vi "Write APD Serial.vi"(8 "error in (no error)":errorcluster, 10 "APD Serial #":string, 11 "APDClass in":refnum<class "APDClass.lvclass">) -> (0 "error out":errorcluster, 3 "APDClass out":refnum<class "APDClass.lvclass">)   [LabVIEW 2020, in "APDClass.lvclass"]
uses:
  APDClass.lvclass
  APDClass.lvclass/APDClass.ctl
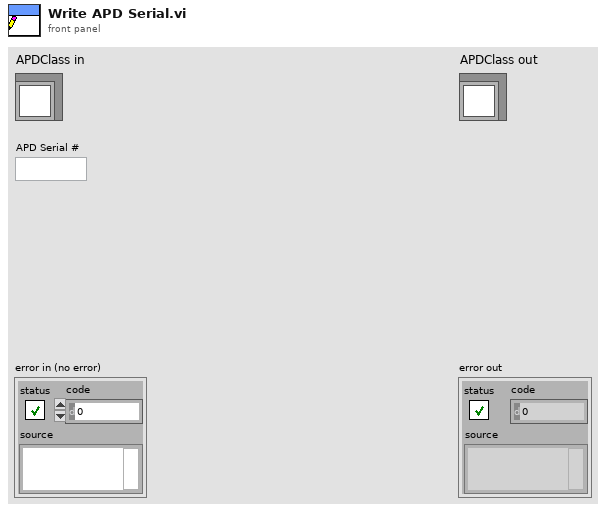
[diagram p1: front panel]
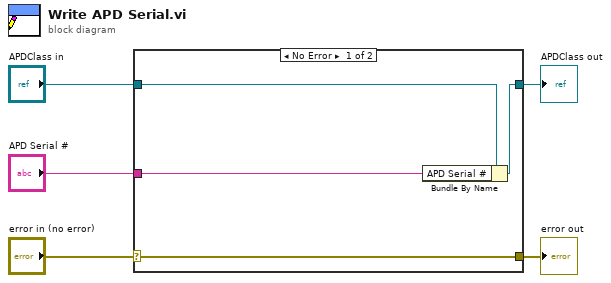
[diagram p0: block diagram]
diagram:
  n1 = case shown="No Error" "error in (no error)" {
    selector: "error in (no error)" -> [w9 w10]
    tunnel: [w9 w10] -> w4
    tunnel: [w7 w11] -> w2
    tunnel: "APDClass in" -> [w8 w11]
    tunnel: "APD Serial #" -> [w6 _]
    frame No Error {
      n2 = Bundle By Name(cluster=w8, "APD Serial #"=w6) -> (w7:refnum<class "APDClass.lvclass">)
    }
    frame Error {
    }
  }
  "error out" <- w4
  "APDClass out" <- w2
